vi "sequencerMCSTopLevel.vi"() -> ()   [LabVIEW 2014]
uses:
  Controls/heinzingerSelect.ctl
  sequencerState.ctl
  Controls/selectTrigger.ctl
  Controls/MCSstate.ctl
  Controls/measVoltState.ctl
  Controls/triggerTypes.ctl
  Controls/triggerEdge.ctl
  OutBits/OutbitsStateControl.ctl
  <vilib>/rvi/Emulation/niFpgaGetClockAttributes.vi
  <vilib>/rvi/Emulation/niFpgaSctlEmulationGetInTimedLoop.vi
  <vilib>/rvi/Emulation/niFpgaEmulationReportErrorSimple.vi
  Trigger/triggerGlobalVars.vi
  <vilib>/rvi/Emulation/niFpgaProcessEmulError.vi
  ScanTrigger/scanTriggerGlobalVars.vi
  StepTrigger/stepTriggerGlobalVars.vi
  sequencerGlobVars.vi
  MCS/MCSGlobalVars.vi
  MeasVolt/measVoltGlobVars.vi
  QueueHandler/queueHandlerGlobals.vi
  HeinzingerControl/heinzingerControlGlobals.vi
  OutBits/OutbitsGlobalVars.vi
  ScanDeviceLogic/scanDeviceGlobalVars.vi
  <vilib>/rvi/Emulation/niFpgaCriticalErrorInLSC.vi
panel:
  out "internalDacAvailable":bool
  in  "ScanDevice":enum16{"internal DAC", "external Python"}(ring)
  in  "scanDevSet":bool
  in  "scanDevTimeout(10ns)":i32
  in  "stepTrigDelay10ns":u32
  in  "softwareStepTrigger":bool
  in  "stepTriggerEdge":T1=enum."true-false"
  in  "stepTriggerTypes":T2
  in  "selectStepTrigger":T3
  in  "scanTrigDelay10ns":u32
  in  "softwareScanTrigger":bool
  in  "scanTriggerEdge":T1=enum."true-false"
  in  "scanTriggerTypes":T2
  in  "selectScanTrigger":T3
  out "nOfCmdsOutbit2":u32
  out "nOfCmdsOutbit1":u32
  out "nOfCmdsOutbit0":u32
  out "OutBitsState":T4
  in  "softwareTrigger":bool
  in  "pause":bool
  in  "stopVoltMeas":bool caption="measVoltStop"
  in  "measVoltCompleteDest":T5(ring)
  in  "dac0VRegister":u32=1572792 format="%024b"
  in  "triggerEdge":T1=enum."true-false"
  out "postAccOffsetVoltState":T6
  in  "triggerTypes":T2=enum."singleHitDelay"
  out "MCSerrorcount":i8
  out "DACQuWriteTimeout":bool
  out "MCSQuWriteTimeout":bool
  out "measVoltState":T7
  out "MCSstate":T8
  in  "nOfBunches":i32
  in  "nOfBins":u32
  in  "trigDelay10ns":u32
  in  "selectTrigger":T3
  in  "hostConfirmsHzOffsetIsSet":bool
  in  "halt":bool
  in  "abort":bool
  in  "cmdByHost":T9
  out "seqState":T9
  in  "timedOutWhileHandshake":bool
  in  "measVoltTimeout(10ns)":i32 caption="measVoltTimeout(25ns)"
  in  "measVoltPulseLength(25ns)":i32
  in  "waitAfterReset(us)":u32 caption="waitForDmm(25nsTicks)"
  in  "waitForKepco(us)":u32
  in  "postAccOffsetVoltControl":T6=enum."loading"
  in  "invertScan":bool
  in  "nOfScans":i32
  in  "nOfSteps":i32
  in  "dacStartRegister20Bit":i32
  in  "dacStepSize20Bit":i32
  in  "VoltOrScaler?":bool
  # "Step Trigger"
  # "Trigger"
  # "Scan Trigger"
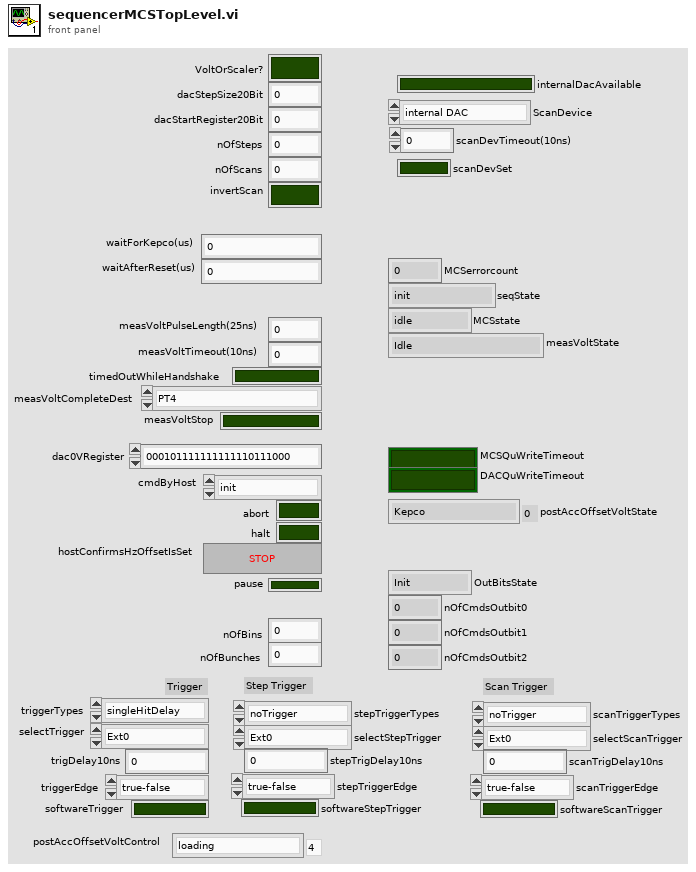
[diagram p1: front panel]
types:
  T1 = typedef "triggerEdge.ctl" = enum8{"either", "false-true", "true-false"}
  T2 = typedef "triggerTypes.ctl" = enum16{"noTrigger", "singleHitDelay", "singleHit", "software", "sweep"}
  T3 = typedef "selectTrigger.ctl" = enum8{"Ext0", "Ext1", "Ext2", "Ext3", "Ext4", "Ext5", "Ext6", "Ext7", "Int0", "Int1", "Int2", "Int3", "Int4", "Int5", "Int6", "Int7"}
  T4 = typedef "OutbitsStateControl.ctl" = enum16{"Init", "Idle", "loading", "listening", "clearing", "error"}
  T5 = enum16{"PT4", "C1D30", "C1D31", "PT4_C1D30", "PT4_C1D31", "PT4_C1D30_C1D31", "C1D30_C1D31"}
  T6 = typedef "heinzingerSelect.ctl" = enum8{"Kepco", "Heinzinger0", "Heinzinger1", "Heinzinger2", "loading"}
  T7 = typedef "measVoltState.ctl" = enum16{"Idle", "sendMeasRequest", "waitUntilDone", "done"}
  T8 = typedef "MCSstate.ctl" = enum16{"idle", "scanning", "done", "error"}
  T9 = typedef "sequencerState.ctl" = enum16{"init", "idle", "measureOffset", "measureTrack", "measComplete", "error"}
  T10 = cluster{"SCLK":refnum<k21>, "CS":refnum<k21>, "MOSI":refnum<k21>, "MISO":refnum<k21>}
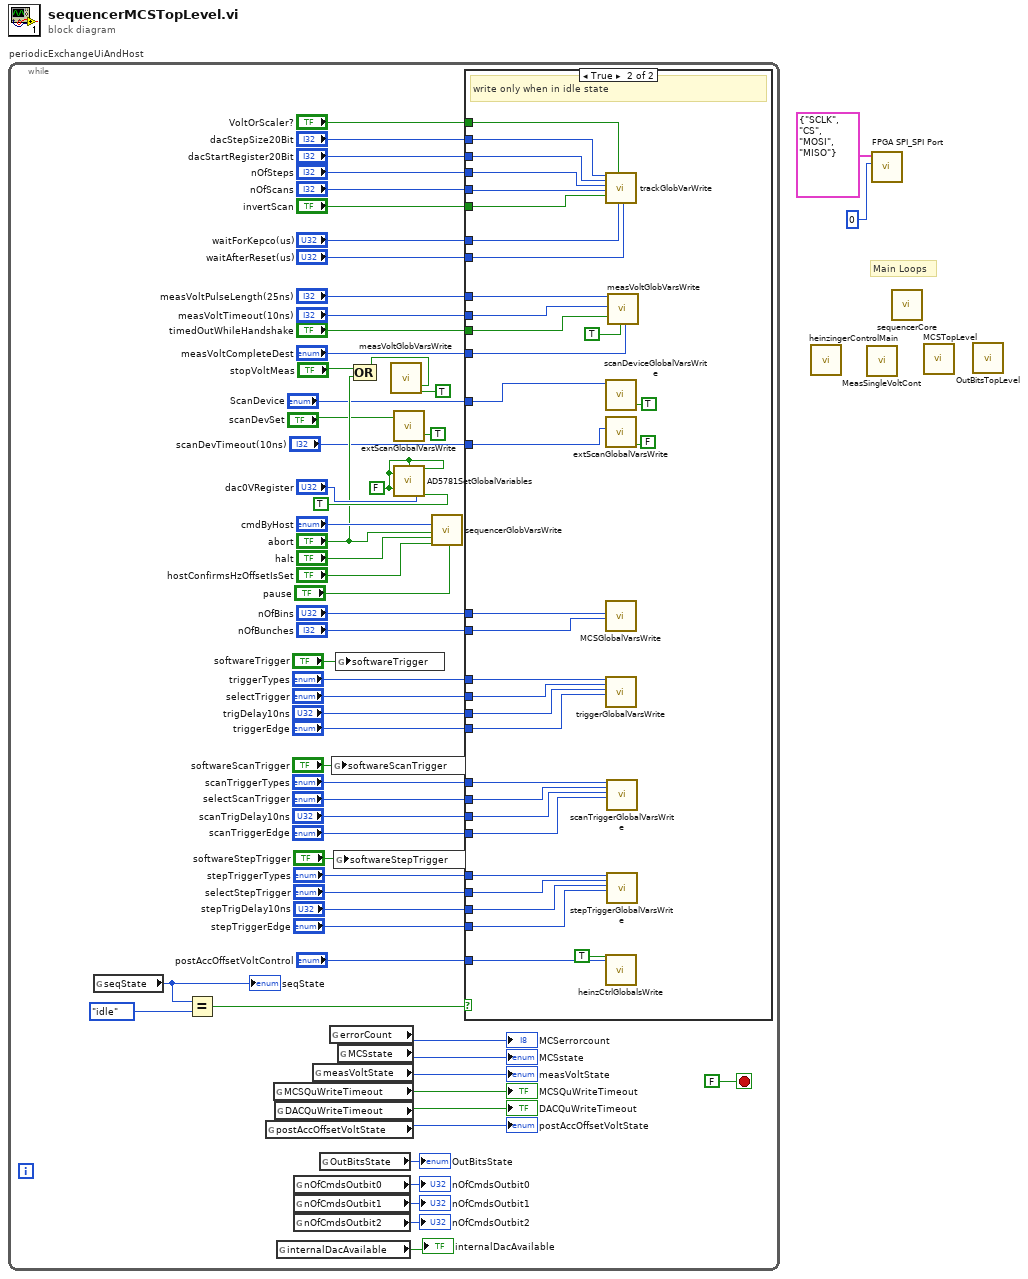
[diagram p0: block diagram]
diagram:
  # "Main Loops"
  n1 = while "periodicExchangeUiAndHost" {
    stop <- FALSE stop-if-true
    w31 = FALSE ("write setDACRegister")
    n2 = global read "sequencerGlobVars.vi" "seqState"() -> (w38:T9)
    "seqState" <- w38
    n3 = Equal?(x=w38, y=sequencerState."idle") -> (x = y?=w61:bool)
    n4 = global read "heinzingerControlGlobals.vi" "postAccOffsetVoltState"() -> (→"postAccOffsetVoltState":T6)
    n5 = global read "queueHandlerGlobals.vi" "MCSQuWriteTimeout"() -> (→"MCSQuWriteTimeout":bool)
    n6 = global read "queueHandlerGlobals.vi" "DACQuWriteTimeout"() -> (→"DACQuWriteTimeout":bool)
    n7 = global read "scanDeviceGlobalVars.vi" "internalDacAvailable"() -> (→"internalDacAvailable":bool)
    n8 = global read "OutbitsGlobalVars.vi" "nOfCmdsOutbit0"() -> (→"nOfCmdsOutbit0":u32)
    n9 = global read "OutbitsGlobalVars.vi" "nOfCmdsOutbit1"() -> (→"nOfCmdsOutbit1":u32)
    n10 = global read "OutbitsGlobalVars.vi" "nOfCmdsOutbit2"() -> (→"nOfCmdsOutbit2":u32)
    n11 = global read "measVoltGlobVars.vi" "measVoltState"() -> (→"measVoltState":T7)
    n12 = global read "OutbitsGlobalVars.vi" "OutBitsState"() -> (→"OutBitsState":T4)
    n13 = global read "MCSGlobalVars.vi" "errorCount"() -> (→"MCSerrorcount":i8)
    n14 = global write "scanTriggerGlobalVars.vi" "softwareScanTrigger"("softwareScanTrigger") -> ()
    n15 = global write "stepTriggerGlobalVars.vi" "softwareStepTrigger"("softwareStepTrigger") -> ()
    n16 = global write "triggerGlobalVars.vi" "softwareTrigger"("softwareTrigger") -> ()
    n17 = global read "MCSGlobalVars.vi" "MCSstate"() -> (→"MCSstate":T8)
    n18 = Compound Arithmetic op=OR("stopVoltMeas", "abort") -> (w27:bool)
    n19 = call "measVoltGlobVarsWrite.vi"("stopVoltMeas"=w27, "writeStopVoltMeas"=TRUE) -> ()  [unwired: 18 in]
    n20 = call "extScanGlobalVarsWrite.vi"("WriteDevSet"=TRUE, "scanDevSet"="scanDevSet") -> ()  [unwired: 10 in]
    n21 = call "AD5781SetGlobalVariables.vi"("write actDACRegister"=w31, "write setDACRegister"=w31, "write DacStateCmdByHost"=w31, "dac0VRegister"="dac0VRegister", "writeSpiGlobals"=w31, "write dac0VRegister"=TRUE) -> ()  [unwired: 14 in]
    n22 = call "sequencerGlobVarsWrite.vi"("cmdByHost"="cmdByHost", "abort"="abort", "halt"="halt", "hostConfirmsHzOffsetIsSet"="hostConfirmsHzOffsetIsSet", "pause"="pause") -> ()  [unwired: 15 in]
    n23 = case shown="True" w61 {
      tunnel: "VoltOrScaler?" -> [_ w95]
      tunnel: "dacStepSize20Bit" -> [_ w94]
      tunnel: "dacStartRegister20Bit" -> [_ w93]
      tunnel: "nOfSteps" -> [_ w92]
      tunnel: "nOfScans" -> [_ w91]
      tunnel: "invertScan" -> [_ w90]
      tunnel: "postAccOffsetVoltControl" -> [_ w81]
      tunnel: "waitForKepco(us)" -> [_ w89]
      tunnel: "waitAfterReset(us)" -> [_ w88]
      tunnel: "measVoltPulseLength(25ns)" -> [_ w87]
      tunnel: "measVoltTimeout(10ns)" -> [_ w86]
      tunnel: "timedOutWhileHandshake" -> [_ w85]
      tunnel: "selectTrigger" -> [_ w79]
      tunnel: "trigDelay10ns" -> [_ w78]
      tunnel: "nOfBins" -> [_ w84]
      tunnel: "nOfBunches" -> [_ w83]
      tunnel: "triggerTypes" -> [_ w80]
      tunnel: "triggerEdge" -> [_ w77]
      tunnel: "measVoltCompleteDest" -> [_ w76]
      tunnel: "scanTriggerTypes" -> [_ w74]
      tunnel: "selectScanTrigger" -> [_ w73]
      tunnel: "scanTrigDelay10ns" -> [_ w72]
      tunnel: "scanTriggerEdge" -> [_ w71]
      tunnel: "stepTriggerTypes" -> [_ w70]
      tunnel: "selectStepTrigger" -> [_ w69]
      tunnel: "stepTrigDelay10ns" -> [_ w68]
      tunnel: "stepTriggerEdge" -> [_ w67]
      tunnel: "ScanDevice" -> [_ w66]
      tunnel: "scanDevTimeout(10ns)" -> [_ w64]
      frame False {
      }
      frame True {
        # "write only when in idle state"
        n24 = call "trackGlobVarWrite.vi"("dacStepSize20Bit"=w94, "dacStartRegister20Bit"=w93, "nOfSteps"=w92, "nOfScans"=w91, "invertScan"=w90, "VoltOrScaler?"=w95, "waitForKepco(us)"=w89, "waitAfterReset(us)"=w88) -> ()  [unwired: 12 in]
        n25 = call "scanDeviceGlobalVarsWrite.vi"("ChooseScanDevice"=TRUE, "ScanDevice"=w66) -> ()  [unwired: 10 in]
        n26 = call "extScanGlobalVarsWrite.vi"("WriteDevSet"=FALSE, "scanDevTimeout(10ns)"=w64) -> ()  [unwired: 10 in]
        n27 = call "MCSGlobalVarsWrite.vi"("nOfBins"=w84, "nOfBunches"=w83) -> ()  [unwired: 18 in]
        n28 = call "triggerGlobalVarsWrite.vi"("triggerTypes"=w80, "selectTrigger"=w79, "delay_10ns_ticks"=w78, "triggerEdge"=w77) -> ()  [unwired: 16 in]
        n29 = call "heinzCtrlGlobalsWrite.vi"("w_postAccOffsetVoltControl"=TRUE, "postAccOffsetVoltControl"=w81) -> ()  [unwired: 26 in]
        n30 = call "scanTriggerGlobalVarsWrite.vi"("scanTriggerTypes"=w74, "selectScanTrigger"=w73, "scan_trig_delay_10ns_ticks"=w72, "scanTriggerEdge"=w71) -> ()  [unwired: 16 in]
        n31 = call "stepTriggerGlobalVarsWrite.vi"("stepTriggerTypes"=w70, "selectStepTrigger"=w69, "step_trig_delay_10ns_ticks"=w68, "stepTriggerEdge"=w67) -> ()  [unwired: 16 in]
        n32 = call "measVoltGlobVarsWrite.vi"("measVoltPulseLength(25ns)"=w87, "measVoltTimeout(10ns)"=w86, "timedOutWhileHandshake"=w85, "writeMeasVoltCompleteDest"=TRUE, "measVoltCompleteDest"=w76) -> ()  [unwired: 15 in]
      }
    }
  }
  n33 = call "heinzingerControlMain.vi"() -> ()  [unwired: 3 in]
  n34 = call "MeasSingleVoltCont.vi"() -> ()  [unwired: 12 in]
  n35 = call "FPGA SPI_SPI Port.vi"("Port"=i8 0, "FPGA IO"=T10 {"SCLK"="SCLK", "CS"="CS", "MOSI"="MOSI", "MISO"="MISO"}) -> ()  [unwired: 10 in]
  n36 = call "sequencerCore.vi"() -> ()  [unwired: 12 in]
  n37 = call "MCSTopLevel.vi"() -> ()  [unwired: 20 in]
  n38 = call "OutBitsTopLevel.vi"() -> ()  [unwired: 12 in]
